vi "Receive_Monitor.vi"(0 "UDP connection ID":refnum<k16>, 11 "error out 2":errorcluster) -> (4 "UDP connection ID out":refnum<k16>, 6 "MonitorBlock":dbl[](array[numeric])=[79.0, 79.0, 0.0, 0.0, 0.0, 0.0, 0.0, 0.0, 0.0, 0.0, 0.0, 0.0, 0.0, 0.0, 0.0, 0.0, 0.0, 0.0, 0.0, 0.0, 0.0, 0.0, 0.0, 0.0, 0.0, 0.0, 0.0, 0.0, 0.0, 0.0, 0.0, 0.0, 0.0, 0.0, 0.0, 0.0, 0.0, 0.0, 0.0, 0.0, 0.0, 0.0, 0.0, 0.0, 0.0, 0.0, 0.0, 0.0, 0.0, 0.0, 0.0, 0.0, 0.0, 0.0, 0.0, 0.0, 0.0, 0.0, 0.0, 0.0, 0.0, 0.0, 0.0, 0.0, 0.0, 0.0, 0.0, 0.0, 0.0, 0.0, 0.0, 0.0, 0.0, 0.0, 0.0, 0.0, 0.0, 0.0, 0.0, 0.0, 0.0, 0.0, 0.0, 0.0, 0.0, 0.0, 0.0, 0.0, 0.0, 0.0, 0.0, 0.0, 0.0, 0.0, 0.0, 0.0] caption="Monitor Data", 15 "error out":errorcluster)   [LabVIEW 2017]
panel:
  out "data out":string
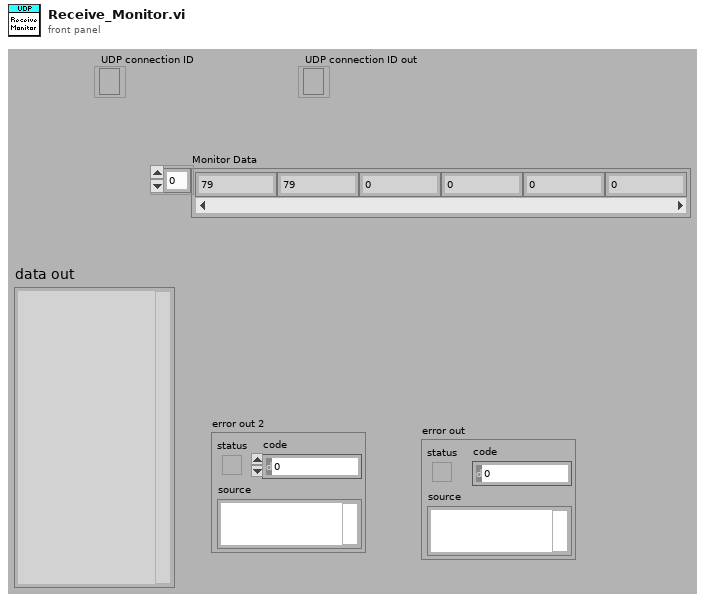
[diagram p1: front panel]
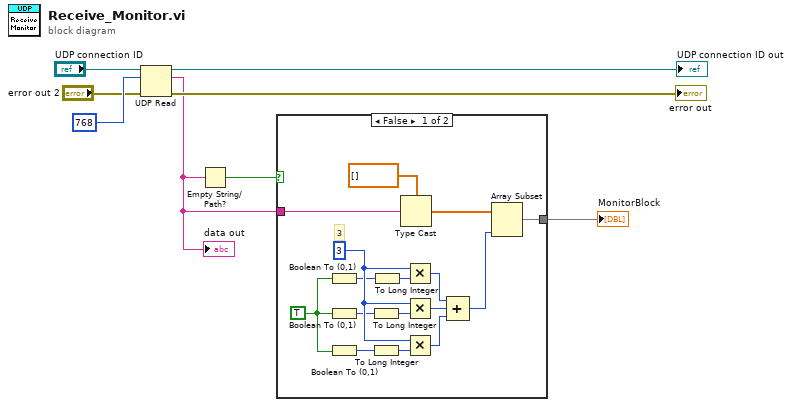
[diagram p0: block diagram]
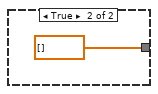
[diagram p2: hidden frame]
diagram:
  n1 = UDP Read(connection ID="UDP connection ID", max size (548)=768, 8:"error out 2") -> (data out=w1:string, error out=→"error out":errorcluster, 3:→"UDP connection ID out":refnum<k16>)  [unwired: 1 in, 2 out]
  "data out" <- w1
  n2 = Empty String/Path?(string/path=w1) -> (empty?=w8:bool)
  n3 = case shown="False" w8 {
    tunnel: w1 -> [w23 _]
    tunnel: [w22 dbl[] []] -> w2
    frame False {
      w21 = TRUE ("Axis3")
      w20 = 3 ("x")
      # "3"
      n4 = Boolean To (0,1)(Boolean=w21) -> (0, 1=w13:i16)
      n5 = Boolean To (0,1)(Boolean=w21) -> (0, 1=w11:i16)
      n6 = Boolean To (0,1)(Boolean=w21) -> (0, 1=w9:i16)
      n7 = To Long Integer(number=w11) -> (32bit integer=w14:i32)
      n8 = To Long Integer(number=w9) -> (32bit integer=w10:i32)
      n9 = To Long Integer(number=w13) -> (32bit integer=w12:i32)
      n10 = Type Cast(type=dbl[] [], x=w23) -> (*(type *) &x=w15:dbl[])
      n11 = Multiply(x=w20, y=w12) -> (x*y=w19:i32)
      n12 = Multiply(x=w20, y=w14) -> (x*y=w18:i32)
      n13 = Multiply(x=w20, y=w10) -> (x*y=w17:i32)
      n14 = Compound Arithmetic op=unknown(w19, w18, w17) -> (w16:i32)
      n15 = Array Subset(array=w15, length=w16) -> (w22:dbl[])  [unwired: 1 in]
    }
    frame True {
    }
  }
  "MonitorBlock" <- w2
